vi "Decimal to Hex Converter.vi"(10 "Decimal":u16) -> (2 "String":string)   [LabVIEW 2017]
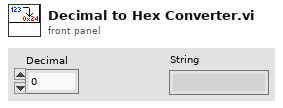
[diagram p1: front panel]
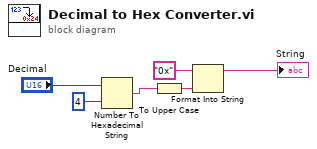
[diagram p0: block diagram]
diagram:
  n1 = Number To Hexadecimal String(1:i16 4 ("width (-)"), 2:"Decimal") -> (0:w4:string)
  n2 = To Upper Case(1:w4) -> (0:w1:string)
  n3 = Format Into String(initial string="0x", w1) -> (resulting string=→"String":string)  [unwired: 2 in, 1 out]
